vi "Mathematical interpolation.vi"(10 "Input data":dbl[][](array[numeric]), 11 "method":i32) -> (2 "Interpolated Data":dbl[][](array[numeric]), 3 "1D Interpolation Graph":cluster{"yi":dbl[], "ramp data":dbl[]}[](graph))   [LabVIEW 2017]
uses:
  <vilib>/Analysis/1siggen.llb/Ramp Pattern by Delta.vi
  <vilib>/gmath/NI_Gmath.lvlib
  <vilib>/Analysis/NI_AALBase.lvlib
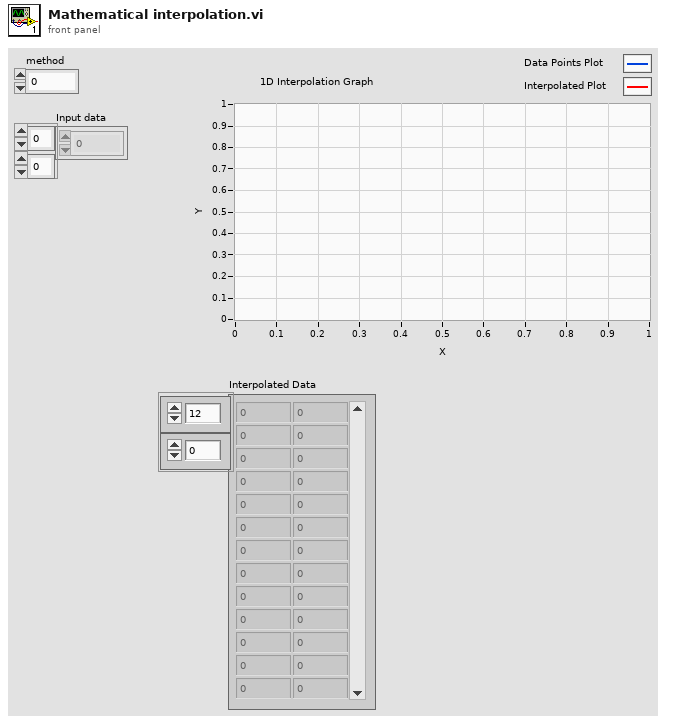
[diagram p1: front panel]
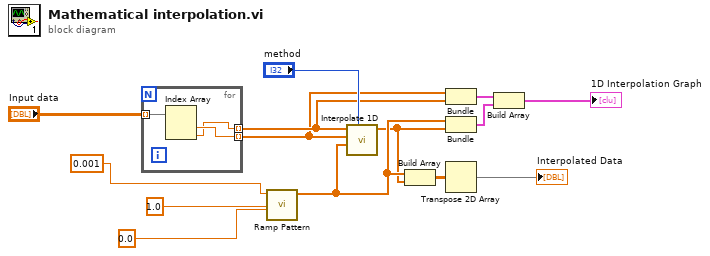
[diagram p0: block diagram]
diagram:
  n1 = for {
    tunnel: [w15] -> w4 mode=indexing
    tunnel: [w16] -> w3 mode=indexing
    tunnel: "Input data" -> [w17] mode=indexing
    n2 = Index Array(array=w17) -> (element #1=w16:dbl, element #2=w15:dbl)  [unwired: 2 in]
  }
  n3 = call-poly <vilib>:"Ramp Pattern.vi"("start"=0.0, "end"=1.0, "delta"=0.001) -> ("Ramp Pattern"=w7:dbl[])  [unwired: 6 in, 2 out]
  n4 = call <vilib>:"Interpolate 1D.vi"("method"="method", "xi"=w7, "X"=w3, "Y"=w4) -> ("yi"=w6:dbl[])  [unwired: 5 in, 2 out]
  n5 = Build Array(w7, w6) -> (w5:dbl[][])
  n6 = Bundle(w3, w4) -> (w2:cluster{dbl[], dbl[]})  [unwired: 1 in]
  n7 = Bundle("Ramp Pattern"=w7, "yi"=w6) -> (w1:cluster{"Ramp Pattern":dbl[], "yi":dbl[]})  [unwired: 1 in]
  n8 = Transpose 2D Array(2D array=w5) -> (transposed array=→"Interpolated Data":dbl[][])
  n9 = Build Array(w2, w1) -> (→"1D Interpolation Graph":cluster{"Ramp Pattern":dbl[], "yi":dbl[]}[])
